vi "外观 1.vi"(0 "Data In":T5=enum."采配水" caption="数据输入", 2 "Display State In":T3 caption="显示状态输入", 3 "Container State":T4 caption="容器状态") -> (6 "Data Out":T5=enum."采配水" caption="数据输出", 7 "Display State Out":T3 caption="显示状态输出", 8 "Action":T2 caption="动作")   [LabVIEW 2016, in "运维调试菜单.xctl"]
uses:
  <vilib>/_xctls/Container State.ctl
  <vilib>/_xctls/Action.ctl
  <vilib>/_xctls/XControlSupport.lvlib
panel:
  in  "单选按钮":T1
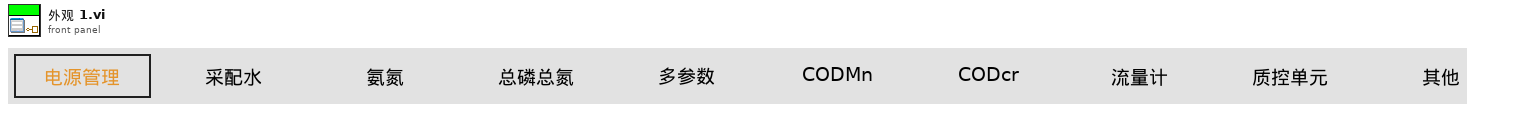
[diagram p1: front panel]
types:
  T1 = typedef "运维调试菜单.xctl/控件外观.ctl" = enum32{"电源管理", "采配水", "氨氮", "总磷总氮", "多参数", "CODMn", "CODcr", "流量计", "质控单元", "其他"}
  T2 = typedef "XControlSupport.lvlib/Action.ctl" = cluster{"Data Changed?":bool, "State Changed?":bool, "Action Name":string}
  T3 = typedef "运维调试菜单.xctl/状态 1.ctl" = cluster{"采配水禁用":enum16{"Enabled", "Disabled", "Disabled and Grayed Out"}, "CODMn禁用":enum16{"Enabled", "Disabled", "Disabled and Grayed Out"}, "CODcr禁用":enum16{"Enabled", "Disabled", "Disabled and Grayed Out"}, "氨氮禁用":enum16{"Enabled", "Disabled", "Disabled and Grayed Out"}, "总磷总氮禁用":enum16{"Enabled", "Disabled", "Disabled and Grayed Out"}, "质控单元禁用":enum16{"Enabled", "Disabled", "Disabled and Grayed Out"}, "流量计禁用":enum16{"Enabled", "Disabled", "Disabled and Grayed Out"}, "电源管理禁用":enum16{"Enabled", "Disabled", "Disabled and Grayed Out"}, "其他禁用":enum16{"Enabled", "Disabled", "Disabled and Grayed Out"}, "多参数禁用":enum16{"Enabled", "Disabled", "Disabled and Grayed Out"}}
  T4 = typedef "XControlSupport.lvlib/Container State.ctl" = cluster{"Indicator?":bool, "Run Mode?":bool, " Refnum":refnum<vi>}
  T5 = typedef "运维调试菜单.xctl/数据 1.ctl" = enum16{"电源管理", "采配水", "氨氮", "总磷总氮", "多参数", "CODMn", "CODcr", "流量计", "质控单元", "其他"}
  T6 = enum16{"Enabled", "Disabled", "Disabled and Grayed Out"}
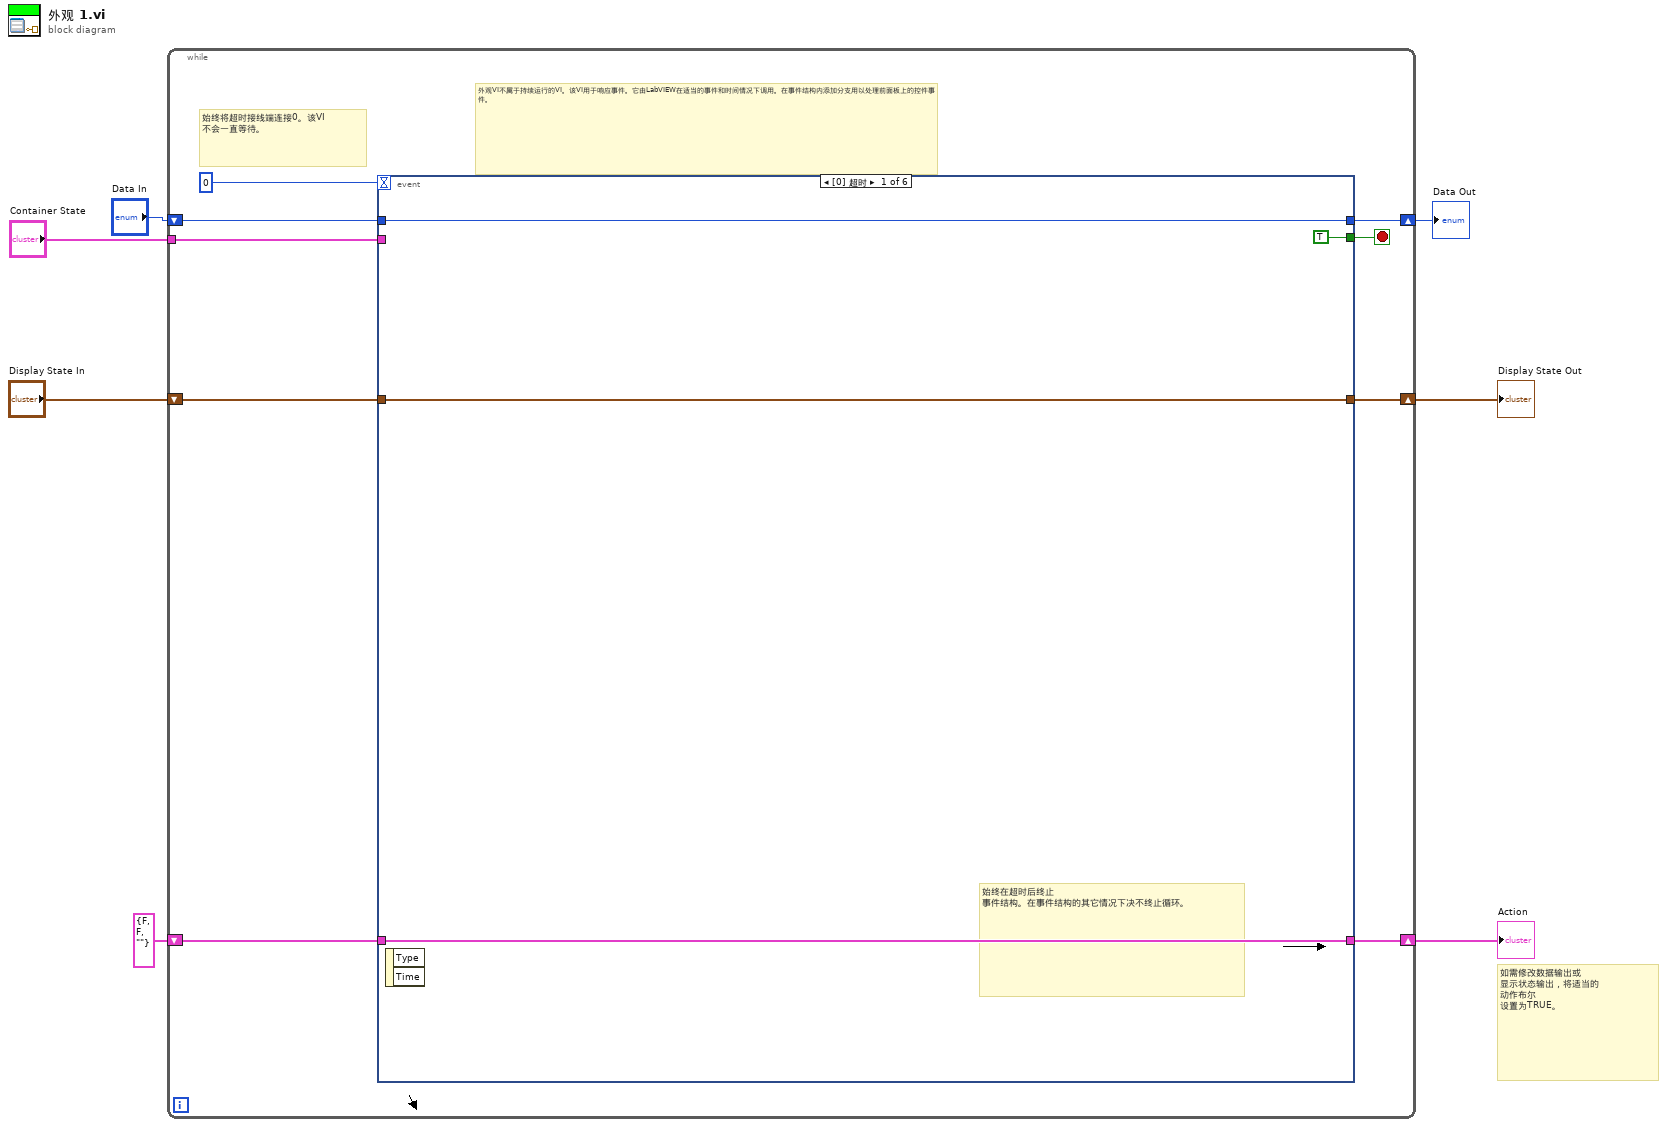
[diagram p0: block diagram]
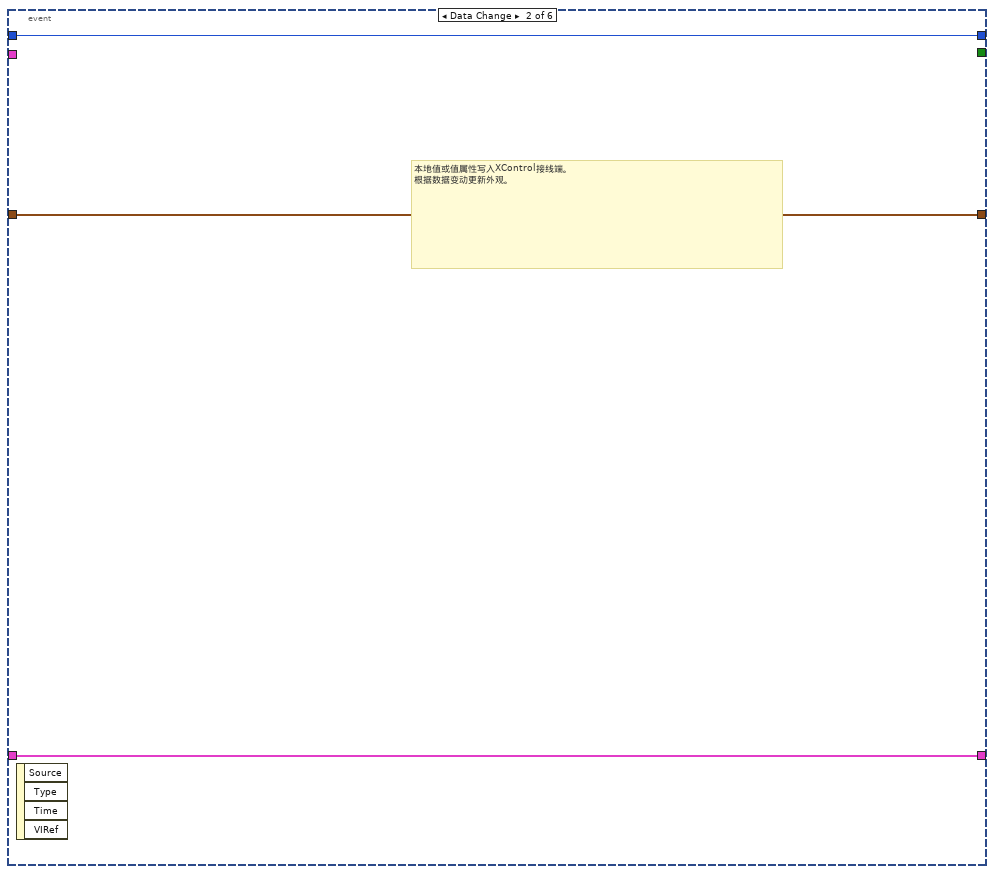
[diagram p2: hidden frame]
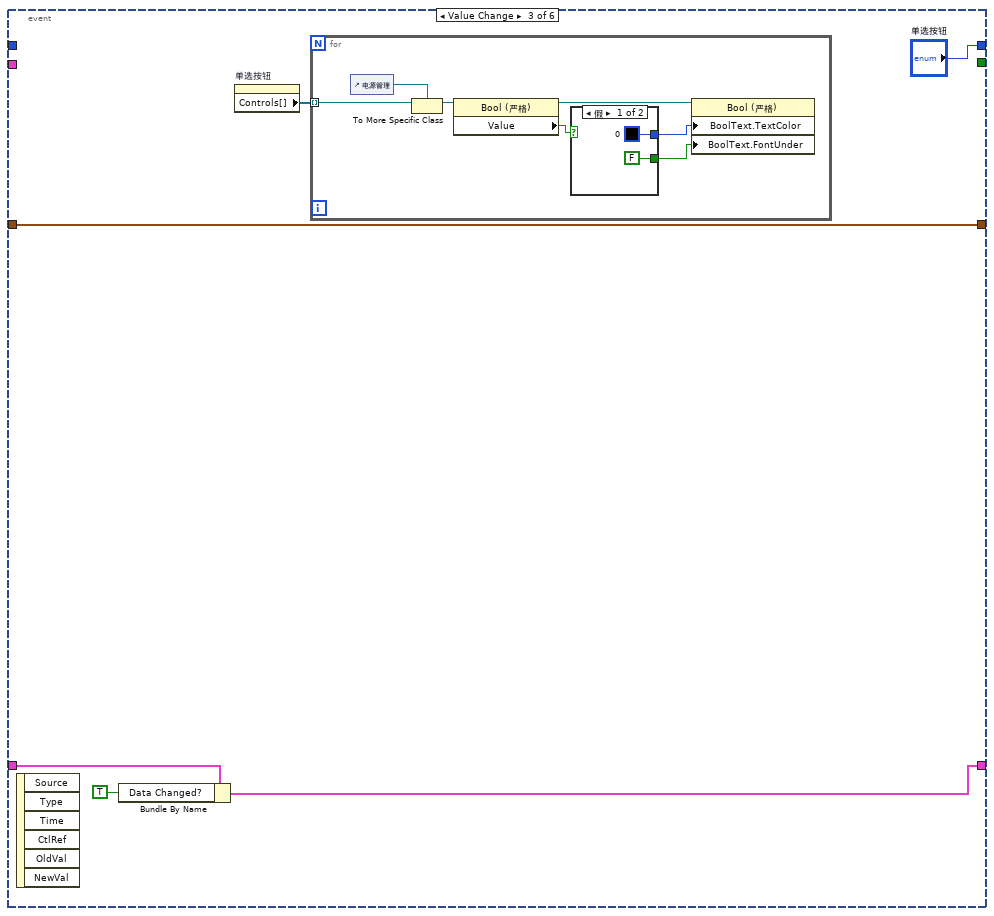
[diagram p3: hidden frame]
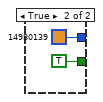
[diagram p4: hidden frame]
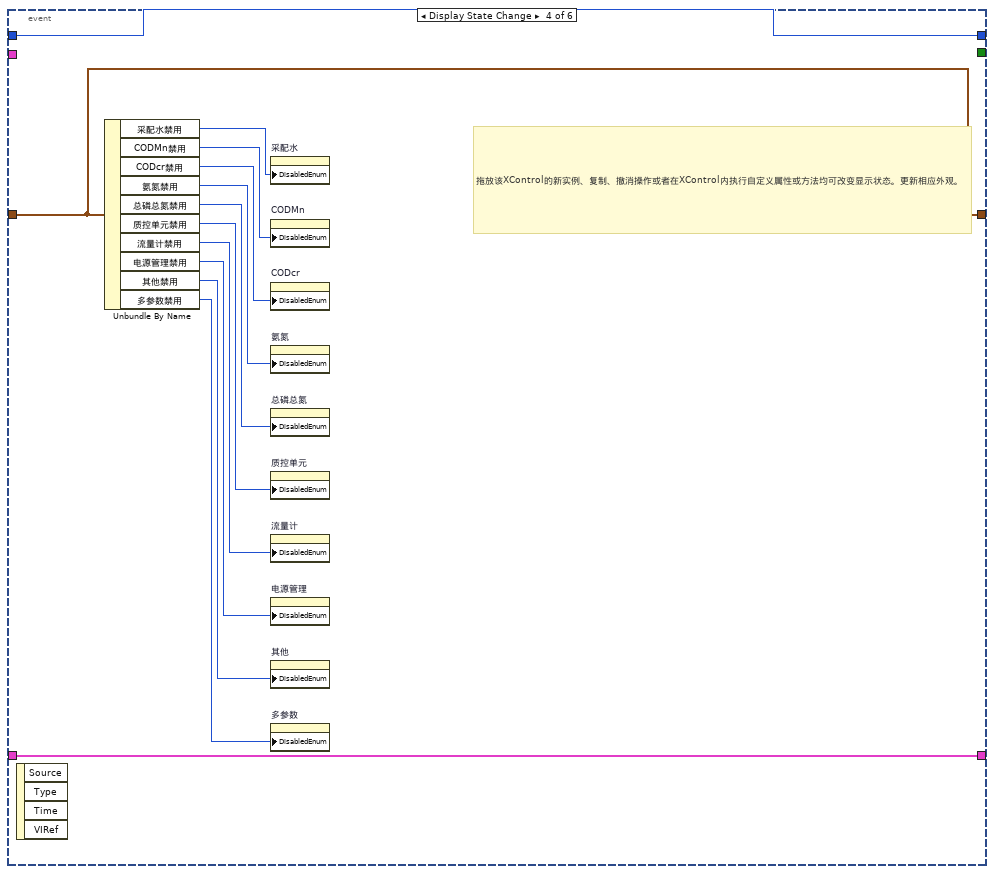
[diagram p5: hidden frame]
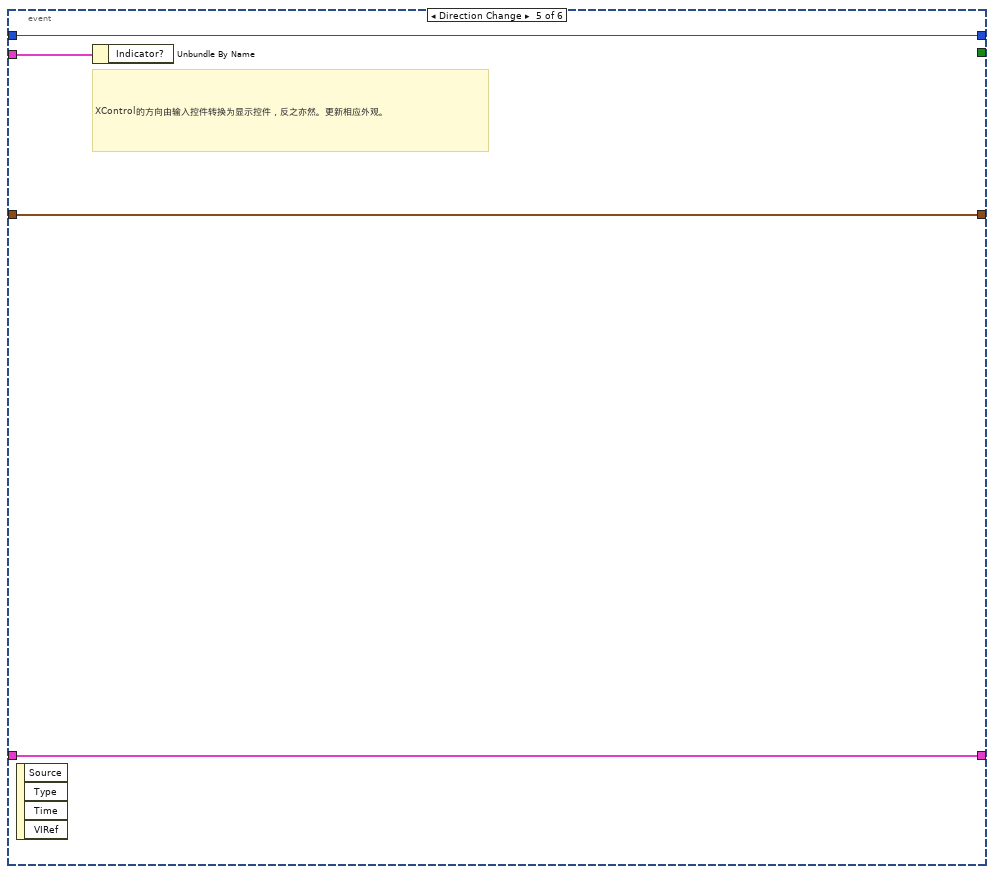
[diagram p6: hidden frame]
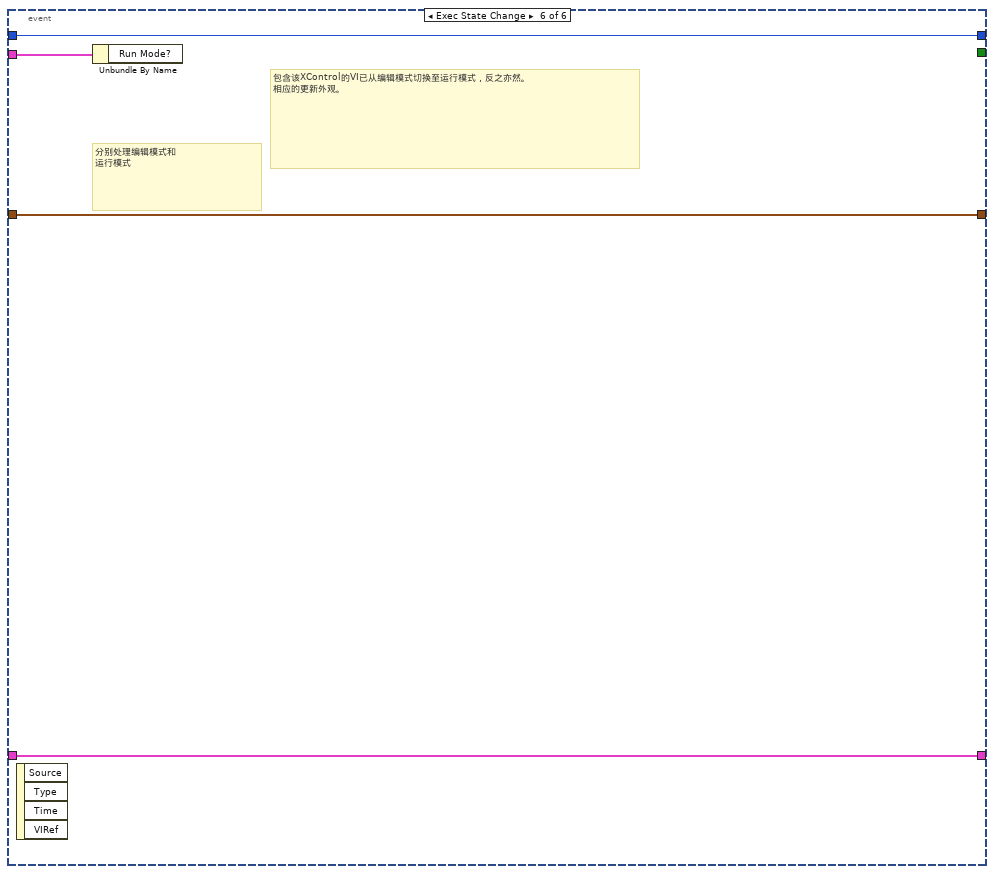
[diagram p7: hidden frame]
diagram:
  # "如需修改数据输出或\n显示状态输出，将适当的\n动作布尔\n设置为TRUE。"
  n1 = while {
    shift-right: [w15] -> w4
    shift-left: "Display State In" -> [w16]
    tunnel: "Container State" -> [w12]
    shift-right: [w10] -> w7
    shift-left: "Data In" -> [w11]
    shift-right: [w8] -> w2
    shift-left: T2 {"Data Changed?"=FALSE, "State Changed?"=FALSE, "Action Name"=""} ("Action") -> [w9]
    stop <- w14 stop-if-true
    # "外观VI不属于持续运行的VI。该VI用于响应事件。它由LabVIEW在适当的事件和时间情况下调用。在事件结构内添加分支用以处理前面板上的控件事件。"
    # "始终将超时接线端连接0。该VI\n不会一直等待。"
    n2 = event shown="[0] 超时" {
      selector: _ -> [_ _ _ _ _ _]
      dyn-events: _ -> [_ _ _ _ _ _]
      timeout: 0 -> [_ _ _ _ _ _]
      tunnel: w16 -> [w18 w22 w29 w44 w56 w60]
      tunnel: [w18 w22 w29 w44 w56 w60] -> w15
      tunnel: [TRUE _ _ _ _ _] -> w14
      tunnel: w12 -> [_ _ _ _ w57 w61]
      tunnel: w11 -> [w17 w23 _ w53 w55 w59]
      tunnel: [w17 w23 "单选按钮" w53 w55 w59] -> w10
      tunnel: [w19 w21 w27 w52 w54 w58] -> w8
      tunnel: w9 -> [w19 w21 w28 w52 w54 w58]
      event Timeout {
        # "始终在超时后终止\n事件结构。在事件结构的其它情况下决不终止循环。"
        n3 = event-data() -> ()  [unwired: 1 in, 2 out]
      }
      event Data Change {
        # "本地值或值属性写入XControl接线端。\n根据数据变动更新外观。"
        n4 = event-data() -> ()  [unwired: 1 in, 4 out]
      }
      event Value Change {
        n5 = event-data() -> ()  [unwired: 1 in, 6 out]
        n6 = Bundle By Name(cluster=w28, "Data Changed?"=TRUE) -> (w27:T2)
        n7 = property on="单选按钮" class="RadioBtnsControl (严格)"() -> ("Controls[]"=w24:refnum<vi>[])  [unwired: 2 in, 2 out]
        n8 = for {
          tunnel: w24 -> [w36] mode=indexing
          n9 = control-ref of="电源管理"() -> (w35:refnum<vi>)
          n10 = To More Specific Class(target class=w35, reference=w36) -> (specific class reference=w34:refnum<vi>)  [unwired: 1 in, 1 out]
          n11 = property class="Bool (严格)"(reference=w34) -> (reference out=w33:refnum<vi>, "Value"=w32:bool)  [unwired: 1 in, 1 out]
          n12 = case shown="假" w32 {
            tunnel: [u32 0 u32 14980139] -> w31
            tunnel: [FALSE ("布尔文本.字体:下划线") TRUE ("布尔文本.字体:下划线")] -> w30
            frame False {
            }
            frame True {
            }
          }
          n13 = property class="Bool (严格)"(reference=w33, "BoolText.TextColor"=w31, "BoolText.FontUnder"=w30) -> ()  [unwired: 1 in, 2 out]
        }
      }
      event Display State Change {
        # "拖放该XControl的新实例、复制、撤消操作或者在XControl内执行自定义属性或方法均可改变显示状态。更新相应外观。"
        n14 = event-data() -> ()  [unwired: 1 in, 4 out]
        n15 = Unbundle By Name(w44) -> ("采配水禁用"=w51:T6, "CODMn禁用"=w50:T6, "CODcr禁用"=w49:T6, "氨氮禁用"=w48:T6, "总磷总氮禁用"=w47:T6, "质控单元禁用"=w46:T6, "流量计禁用"=w43:T6, "电源管理禁用"=w42:T6, "其他禁用"=w45:T6, "多参数禁用"=w41:T6)
        n16 = property on="采配水" class="Bool (严格)"("DisabledEnum"=w51) -> ()  [unwired: 2 in, 2 out]
        n17 = property on="CODMn" class="Bool (严格)"("DisabledEnum"=w50) -> ()  [unwired: 2 in, 2 out]
        n18 = property on="CODcr" class="Bool (严格)"("DisabledEnum"=w49) -> ()  [unwired: 2 in, 2 out]
        n19 = property on="氨氮" class="Bool (严格)"("DisabledEnum"=w48) -> ()  [unwired: 2 in, 2 out]
        n20 = property on="总磷总氮" class="Bool (严格)"("DisabledEnum"=w47) -> ()  [unwired: 2 in, 2 out]
        n21 = property on="质控单元" class="Bool (严格)"("DisabledEnum"=w46) -> ()  [unwired: 2 in, 2 out]
        n22 = property on="流量计" class="Bool (严格)"("DisabledEnum"=w43) -> ()  [unwired: 2 in, 2 out]
        n23 = property on="电源管理" class="Bool (严格)"("DisabledEnum"=w42) -> ()  [unwired: 2 in, 2 out]
        n24 = property on="其他" class="Bool (严格)"("DisabledEnum"=w45) -> ()  [unwired: 2 in, 2 out]
        n25 = property on="多参数" class="Bool (严格)"("DisabledEnum"=w41) -> ()  [unwired: 2 in, 2 out]
      }
      event Direction Change {
        # "XControl的方向由输入控件转换为显示控件，反之亦然。更新相应外观。"
        n26 = event-data() -> ()  [unwired: 1 in, 4 out]
        n27 = Unbundle By Name(w57) -> ()  [unwired: 1 out]
      }
      event Exec State Change {
        # "包含该XControl的VI已从编辑模式切换至运行模式，反之亦然。\n相应的更新外观。"
        # "分别处理编辑模式和\n运行模式"
        n28 = event-data() -> ()  [unwired: 1 in, 4 out]
        n29 = Unbundle By Name(w61) -> ()  [unwired: 1 out]
      }
    }
  }
  "Display State Out" <- w4
  "Data Out" <- w7
  "Action" <- w2
